vi "檔案_速度.vi"() -> ()   [LabVIEW 2015]
panel:
  out "存檔":bool
  in  "全速百分比":u32
  in  "Save Button":bool
  out "Recipe":string
  in  "Exit":bool
  # "Recipe - 馬達速度表(mm/s)"
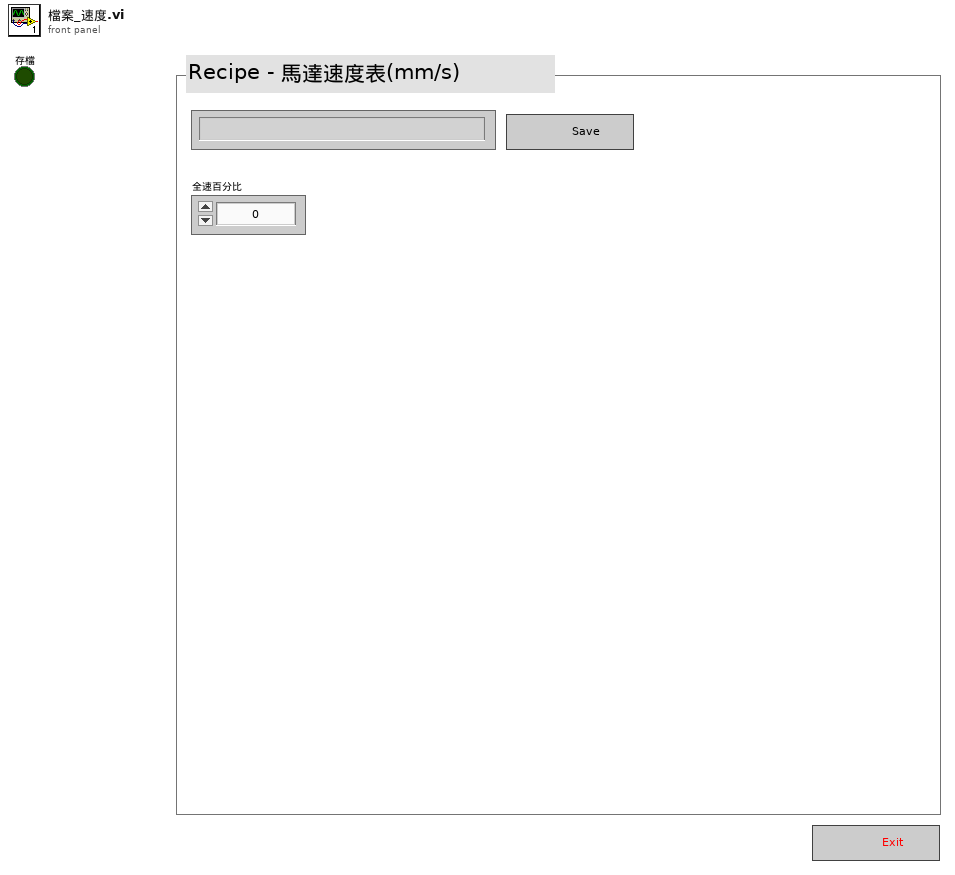
[diagram p1: front panel]
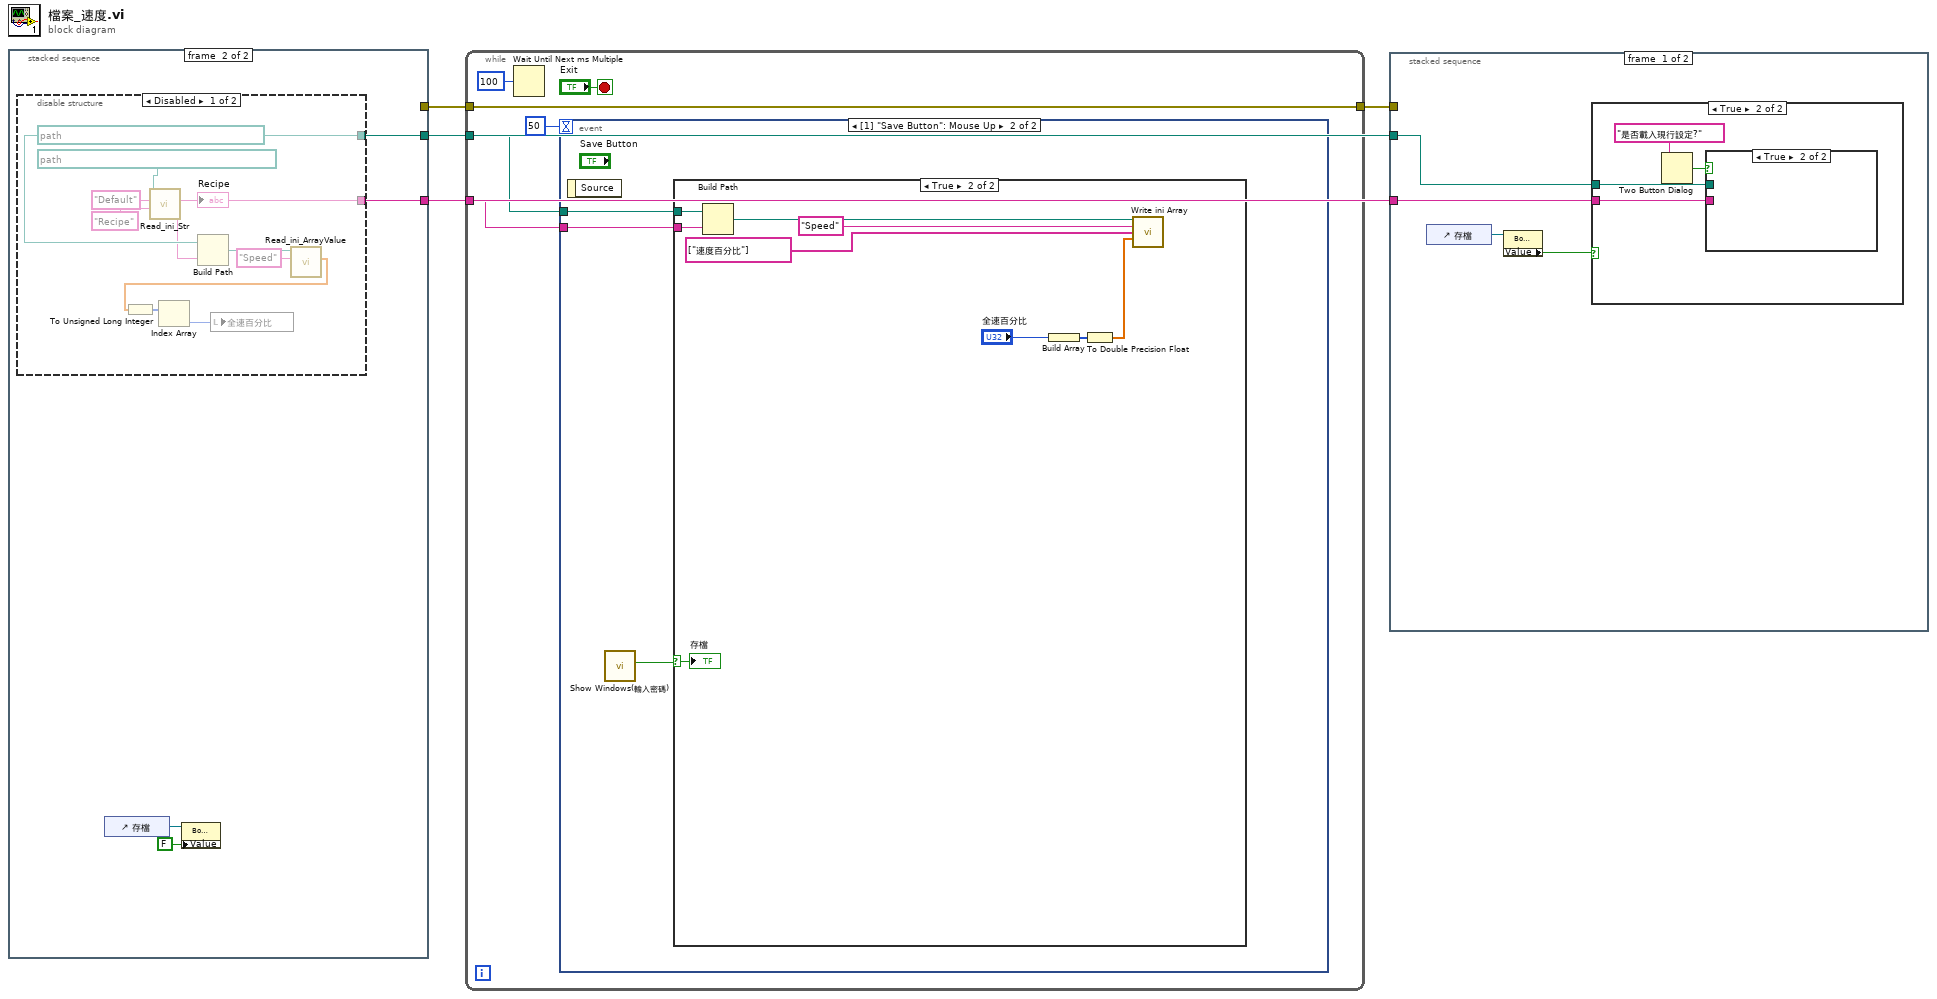
[diagram p0: block diagram]
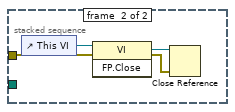
[diagram p4: hidden frame]
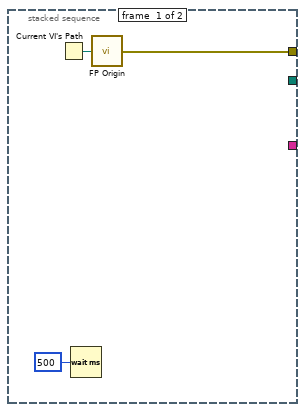
[diagram p5: hidden frame]
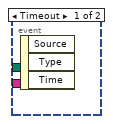
[diagram p7: hidden frame]
diagram:
  n1 = stacked-sequence {
    tunnel: [w6 _] -> w3
    tunnel: [_ w10] -> w1
    tunnel: [_ w11] -> w2
    frame #0 {
      n2 = Current VI's Path() -> (path=w7:path)
      n3 = Wait (ms)(milliseconds to wait=u32 500) -> ()  [unwired: 1 out]
      n4 = call "FP Origin.vi"("vi path"=w7) -> ("error out"=w6:errorcluster)
    }
    frame #1 {
      n5 = disable-structure shown="Disabled" {
        disable-tunnel: [w18 _] -> w11
        disable-tunnel: [w17 _] -> w10
        frame Disabled {
          w18 = path "D:/半自動電檢機 Data/Recipe/Position" ("configuration file path")
          n6 = call "Read_ini_Str.vi"("key"="Recipe", "section"="Default", "configuration file path"=path "D:/半自動電檢機 Data/Recipe/Default.ini") -> ("value"=w17:string)  [unwired: 7 in, 1 out]
          "Recipe" <- w17
          n7 = Build Path(base path=w18, name or relative path=w17) -> (appended path=w16:path)
          n8 = call "Read_ini_ArrayValue.vi"("section"="Speed", "configuration file path"=w16) -> ("ArrayValue"=w14:dbl[])  [unwired: 8 in, 1 out]
          n9 = To Unsigned Long Integer(number=w14) -> (unsigned 32bit integer=w13:u32[])
          n10 = Index Array(array=w13) -> (element=w12:u32)  [unwired: 1 in]
          n11 = local write "全速百分比"(w12) -> ()
        }
        frame Enabled {
        }
      }
      n12 = control-ref of="存檔"() -> (w9:refnum<vi>)
      n13 = property class="Bool (strict)"(reference=w9, "Value"=FALSE) -> ()  [unwired: 1 in, 2 out]
    }
  }
  n14 = while {
    tunnel: w3 -> [w24]
    tunnel: [w24] -> w4
    tunnel: w1 -> [w23]
    tunnel: w2 -> [w22]
    stop <- "Exit" stop-if-true
    n15 = Wait Until Next ms Multiple(millisecond multiple=u32 100) -> ()  [unwired: 1 out]
    n16 = event shown="[1] \"Save Button\": Mouse Up" {
      selector: _ -> [_ _]
      dyn-events: _ -> [_ _]
      timeout: 50 -> [_ _]
      tunnel: w23 -> [_ w30]
      tunnel: w22 -> [_ w29]
      event Timeout {
        n17 = event-data() -> ()  [unwired: 1 in, 3 out]
      }
      event "Save Button": Mouse Up {
        n18 = event-data() -> ()  [unwired: 1 in, 1 out]
        n19 = call "Show Windows(輸入密碼).vi"() -> ("密碼正確"=w28:bool)  [unwired: 10 in, 1 out]
        n20 = case shown="True" w28 {
          selector: w28 -> [_ w31]
          tunnel: w30 -> [_ w39]
          tunnel: w29 -> [_ w38]
          frame False {
          }
          frame True {
            n21 = Build Path(base path=w38, name or relative path=w39) -> (appended path=w37:path)
            n22 = Build Array("全速百分比") -> (w33:u32[])
            n23 = To Double Precision Float(number=w33) -> (double precision float=w32:dbl[])
            n24 = call "Write ini Array.vi"("configuration file path"=w37, "section"="Speed" ("key"), "KeysArray"=string[] ["速度百分比"], "ValueArray"=w32) -> ()  [unwired: 11 in, 1 out]
            "存檔" <- w31
          }
        }
      }
    }
  }
  n25 = stacked-sequence {
    tunnel: w4 -> [_ w51]
    tunnel: w2 -> [w43 _]
    tunnel: w1 -> [w42 _]
    frame #0 {
      n26 = control-ref of="存檔"() -> (w41:refnum<vi>)
      n27 = property class="Bool (strict)"(reference=w41) -> ("Value"=w40:bool)  [unwired: 1 in, 2 out]
      n28 = case shown="True" w40 {
        tunnel: w43 -> [_ w45]
        tunnel: w42 -> [_ w44]
        frame False {
        }
        frame True {
          n29 = Two Button Dialog(message="是否載入現行設定?") -> (T button?=w47:bool)  [unwired: 2 in]
          n30 = case shown="True" w47 {
            tunnel: w45 -> [_ _]
            tunnel: w44 -> [_ _]
            frame False {
            }
            frame True {
            }
          }
        }
      }
    }
    frame #1 {
      n31 = control-ref of="This VI"() -> (w50:refnum<vi>)
      n32 = invoke class="VI" method="FP.Close"(reference=w50, error in=w51) -> (reference out=w49:refnum<vi>, error out=w48:errorcluster)  [unwired: 1 in, 1 out]
      n33 = Close Reference(reference=w49, error in (no error)=w48) -> ()  [unwired: 1 out]
    }
  }
